vi "NIDMMcontTriggered.vi"() -> ()   [LabVIEW 2014]
uses:
  <instrlib>/niDMM/nidmm.llb/niDMM Slope.ctl
  <instrlib>/niDMM/nidmm.llb/niDMM Trigger.ctl
  <instrlib>/niDMM/nidmm.llb/niDMM Resolution in Digits.ctl
  <instrlib>/niDMM/nidmm.llb/niDMM Function.ctl
  <instrlib>/niDMM/nidmm.llb/niDMM Sample Trigger.ctl
  <instrlib>/niDMM/nidmm.llb/niDMM Configure Measurement Digits.vi
panel:
  in  "Function":T1
  in  "Resolution in Digits":T2=5.5 items=["3 1/2"=3.5, "4 1/2"=4.5, "5 1/2"=5.5, "6 1/2"=6.5, "7 1/2"=7.5]
  in  "Range":dbl=10.0 format="%.2p"
  in  "stop":bool
  out "Measurements":dbl[](graph)
  in  "Trigger Source":T3=enum."External"
  in  "Slope":T4=enum."Falling Edge"
  in  "Device Name":refnum<k15>="Dev1"
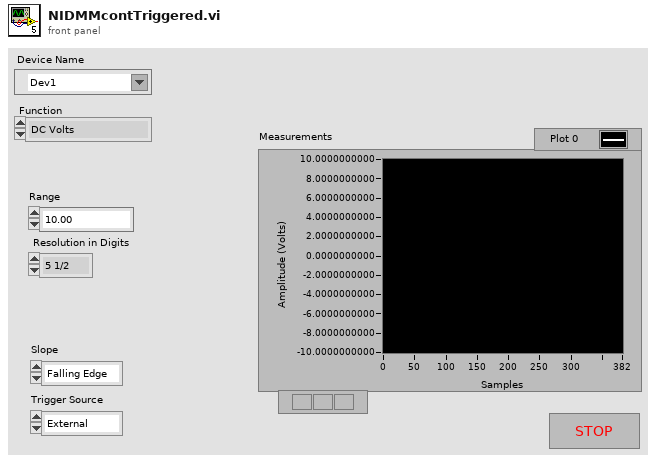
[diagram p1: front panel]
types:
  T1 = typedef "niDMM Function.ctl" = enum16{"DC Volts", "AC Volts", "DC Current", "AC Current", "2-wire Resistance", "4-wire Resistance", "Diode", "Frequency", "Period", "AC Volts DC Coupled", "Capacitance", "Inductance", "Temperature"}
  T2 = typedef "niDMM Resolution in Digits.ctl" = dbl
  T3 = typedef "niDMM Trigger.ctl" = enum16{"Immediate", "External", "TTL 0", "TTL 1", "TTL 2", "TTL 3", "TTL 4", "TTL 5", "TTL 6", "Software", "TTL 7", "PXI Star", "LBR Trig 1", "Aux Trig 1"}
  T4 = typedef "niDMM Slope.ctl" = enum16{"Rising Edge", "Falling Edge"}
  T5 = typedef "niDMM Sample Trigger.ctl" = enum16{"Immediate", "External", "TTL 0", "TTL 1", "TTL 2", "TTL 3", "TTL 4", "TTL 5", "TTL 6", "Interval", "Software", "TTL 7", "PXI Star", "LBR Trig 1", "Aux Trig 1"}
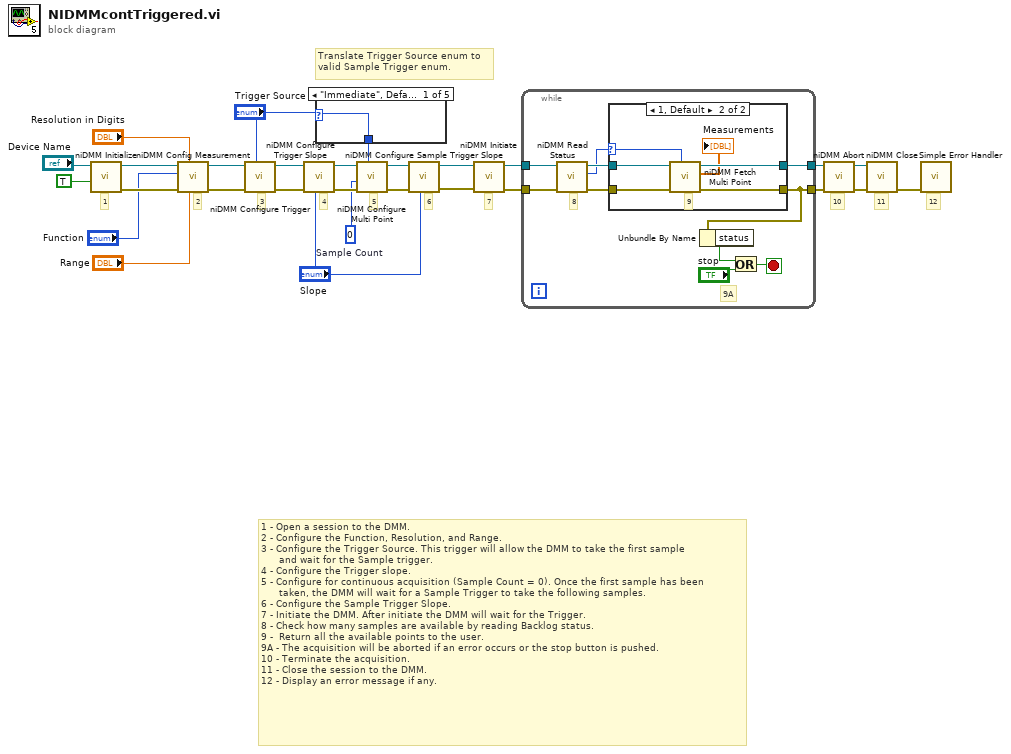
[diagram p0: block diagram]
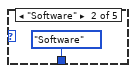
[diagram p3: hidden frame]
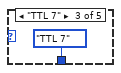
[diagram p4: hidden frame]
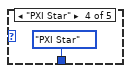
[diagram p5: hidden frame]
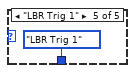
[diagram p6: hidden frame]
diagram:
  w11 = 0  # Sample Count
  # "4"
  # "12"
  # "10"
  # "6"
  # "11"
  # "5"
  # "7"
  # "Translate Trigger Source enum to\nvalid Sample Trigger enum."
  # "3"
  # "2"
  # "1"
  # "1 - Open a session to the DMM.\n2 - Configure the Function, Resolution, and Range.\n3 - Configure the Trigger Source. This trigger will allow the DMM to take the first sample\n      and wait for the Sample trigger.\n4 - Configure the Trigger slope.\n5 - Configure for continuous acquisition (Sample Count = 0). Once the first sample has been\n      taken, the DMM will wait for a Sample Trigger to take the following samples.\n6 - Configure the Sample Trigger Slope.\n7 - Initiate the DMM. After initiate the DMM will wait for the Trigger.\n8 - Check how many samples are available by reading Backlog status.  \n9 -  Return all the available points to the user. \n9A - The acquisition will be aborted if an error occurs or the stop button is pushed.\n10 - Terminate the acquisition.\n11 - Close the session to the DMM.\n12 - Display an error message if any."
  n1 = call <instrlib>:"niDMM Initialize.vi"("Reset"=TRUE, "Instrument Descriptor"="Device Name") -> ("error out"=w27:errorcluster, "instrument handle out"=w28:refnum<k15>)  [unwired: 8 in]
  n2 = call-poly <instrlib>:"niDMM Config Measurement.vi"("Range"="Range", "Resolution in Digits"="Resolution in Digits", "error in (no error)"=w27, "Function"="Function", "instrument handle"=w28) -> ("error out"=w19:errorcluster, "instrument handle out"=w20:refnum<k15>)  [unwired: 5 in]
  n3 = call <instrlib>:"niDMM Configure Trigger.vi"("Trigger Source"="Trigger Source", "error in (no error)"=w19, "instrument handle"=w20) -> ("error out"=w17:errorcluster, "instrument handle out"=w18:refnum<k15>)  [unwired: 7 in]
  n4 = call <instrlib>:"niDMM Configure Trigger Slope.vi"("Slope"="Slope", "error in (no error)"=w17, "instrument handle"=w18) -> ("error out"=w15:errorcluster, "instrument handle out"=w16:refnum<k15>)  [unwired: 7 in]
  n5 = case shown="\"Immediate\", Default" "Trigger Source" {
    selector: "Trigger Source" -> [w29 _ _ _ _]
    tunnel: [w29 niDMM_Sample_Trigger."Software" ("Sample Trigger") niDMM_Sample_Trigger."TTL 7" ("Sample Trigger") niDMM_Sample_Trigger."PXI Star" ("Sample Trigger") niDMM_Sample_Trigger."LBR Trig 1" ("Sample Trigger")] -> w5
    frame "Immediate", Default {
    }
    frame "Software" {
    }
    frame "TTL 7" {
    }
    frame "PXI Star" {
    }
    frame "LBR Trig 1" {
    }
  }
  n6 = call <instrlib>:"niDMM Configure Multi Point.vi"("Sample Trigger"=w5, "error in (no error)"=w15, "Sample Count"=w11, "instrument handle"=w16) -> ("error out"=w13:errorcluster, "instrument handle out"=w14:refnum<k15>)  [unwired: 6 in]
  n7 = call <instrlib>:"niDMM Configure Sample Trigger Slope.vi"("Slope"="Slope", "error in (no error)"=w13, "instrument handle"=w14) -> ("error out"=w7:errorcluster, "instrument handle out"=w4:refnum<k15>)  [unwired: 7 in]
  n8 = call <instrlib>:"niDMM Initiate.vi"("error in (no error)"=w7, "instrument handle"=w4) -> ("error out"=w26:errorcluster, "instrument handle out"=w25:refnum<k15>)  [unwired: 8 in]
  n9 = while {
    tunnel: [w43] -> w8
    tunnel: w25 -> [w39]
    tunnel: [w35] -> w9
    tunnel: w26 -> [w38]
    stop <- w40 stop-if-true
    # "9A"
    # "8"
    n10 = call <instrlib>:"niDMM Read Status.vi"("error in (no error)"=w38, "instrument handle"=w39) -> ("error out"=w37:errorcluster, "Backlog"=w34:i32, "instrument handle out"=w36:refnum<k15>)  [unwired: 6 in, 1 out]
    n11 = case shown="1, Default" w34 {
      selector: w34 -> [_ w46]
      tunnel: [w45 w51] -> w43
      tunnel: [w44 w49] -> w35
      tunnel: w37 -> [w44 w48]
      tunnel: w36 -> [w45 w47]
      frame 0 {
      }
      frame 1, Default {
        # "9"
        n12 = call <instrlib>:"niDMM Fetch Multi Point.vi"("Number to Fetch"=w46, "error in (no error)"=w48, "instrument handle"=w47) -> ("error out"=w49:errorcluster, "Measurements"=→"Measurements":dbl[], "instrument handle out"=w51:refnum<k15>)  [unwired: 5 in, 1 out]
      }
    }
    n13 = Unbundle By Name(w35) -> ("status"=w42:bool)
    n14 = Or(x=w42, y="stop") -> (x .or. y?=w40:bool)
  }
  n15 = call <instrlib>:"niDMM Abort.vi"("error in (no error)"=w9, "instrument handle"=w8) -> ("error out"=w23:errorcluster, "instrument handle out"=w24:refnum<k15>)  [unwired: 8 in]
  n16 = call <instrlib>:"niDMM Close.vi"("error in (no error)"=w23, "instrument handle"=w24) -> ("error out"=w3:errorcluster)  [unwired: 9 in]
  n17 = call <vilib>:"Simple Error Handler.vi"("error in (no error)"=w3) -> ()  [unwired: 4 in, 5 out]
